vi "Query VIRef with Error Cache.vi"(6 "Reset(F)":bool, 7 "Current Module(\"\" to generate a ID)":string, 8 "Error In (no error)":errorcluster, 9 "Target Module":string="A") -> (0 "error out":errorcluster, 3 "CSM VI Ref":refnum<vi>)   [LabVIEW 2020, in "CSM Mermaid Support.lvlib"]
uses:
  CSM Mermaid Support.lvlib
  <userlib>/_NEVSTOP/Communicable State Machine(CSM)/Communicable State Machine.lvlib
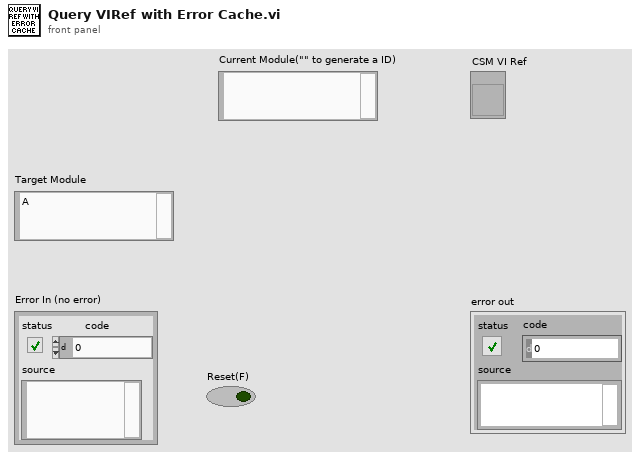
[diagram p1: front panel]
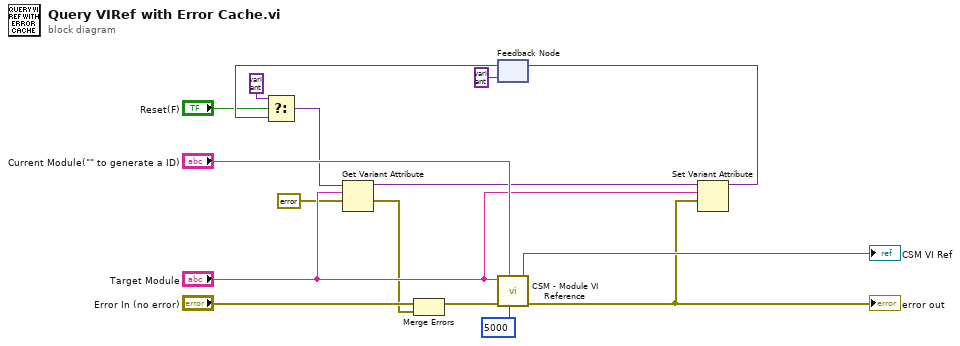
[diagram p0: block diagram]
diagram:
  n1 = feedback #1(variant) -> (w5:variant)
  n2 = Select(t=variant, s="Reset(F)", f=w5) -> (s? t:f=w1:variant)
  n3 = Get Variant Attribute(Variant=w1, name="Target Module", default value (empty Variant)=errorcluster {"status"=FALSE, "code"=0, "source"=""} ("error in (no error)")) -> (duplicate Variant=w12:variant, value=w6:errorcluster)  [unwired: 1 in, 2 out]
  n4 = Merge Errors("Error In (no error)", w6) -> (w7:errorcluster)
  n5 = call <userlib>:"CSM - Module VI Reference.vi"("Response Timeout(-2 using Global Settings)"=5000 ("Response Timeout(5000ms)"), "Current Module(\"\" to generate a ID)"="Current Module(\"\" to generate a ID)", "error in (no error)"=w7, "CSM Name"="Target Module") -> ("error out"=w10:errorcluster, "CSM Module VIRef"=→"CSM VI Ref":refnum<vi>)  [unwired: 6 in]
  "error out" <- w10
  n6 = Set Variant Attribute(Variant=w12, name="Target Module", value=w10) -> (Variant out=w11:variant)  [unwired: 1 in, 2 out]
  n7 = feedback-in #1(w11) -> ()
